vi "DefenderNormalNova.vi"(0 "Tipo de \nmarcador":T1(ring), 1 "Atacando contra?":bool=TRUE, 3 "AI Parameters":T9={"GotoKick"={"Dist do cone a frente"=150.0, "attacker farback"=1500.0, "Perto"=300.0, "min dist to kick"=150.0, "kick eps"=0.0, "Time to transition"=0.05}, "Attacker"={"CC chute"=0.09, "CC passe"=0.045, "Kick Force"=100.0, "ball-robot Kick"=200.0, "ball-robot Pass"=0.3, "drible\nAttk"=FALSE}, "Defender"={"D max"=1700.0, "Vel p/ robô av"=1000.0, "Kick Force"=100.0, "D atk-def"=0.0, "D farback"=0.0, "drible\ndef"=FALSE, "drible\ngoalie"=FALSE}, "Timeout"={"Field/v in x"=6.0, "Dist Robots"=300, "Dist up in y"=300}, "Pose Striker"={"dist"=200.0, "Numeric"=-4.0, "dist 2"=200.0, "drible\nstriker"=FALSE}, "Dist Stop"=300.0, "D ball out"=200, "D central gap "=150.0, "T pass"=0.0, "Force ++"=0.0, "range kick"=0.0, "Chute alto"=TRUE, "Marcador novo"=TRUE, "drible"=FALSE, "D drible"=300.0, "Versão Striker"=enum."Auto", "Defesa"=enum."Barreira", "Marcador"=enum."Marcar Segundo mais perigoso", "Receptor passe"=enum."Auto", "Área"=enum."Quadrada"} {"D drible" format="%#_13g"; "D central gap" format="%#_13g"; "Dist Stop" format="%#_13g"; "Pose Striker"."Numeric" format="%#_13g"; "Defender"."Kick Force" format="%#_13g"; "Defender"."Vel p/ robô av" format="%#_13g"; "Attacker"."ball-robot Kick" format="%#_13g"; "Attacker"."Kick Force" format="%#_13g"; "Attacker"."CC passe" format="%#_13g"; "Attacker"."CC chute" format="%#_13g"; "GotoKick"."kick eps" format="%#_13g"; "GotoKick"."min dist to kick" format="%#_13g"; "GotoKick"."Perto" format="%#_13g"; "GotoKick"."attacker farback" format="%#_13g"; "GotoKick"."Dist do cone a frente" format="%#_13g"}, 4 "IA State Input 2":T10={"our_robots"=[], "enemy_robots"=[], "balls"=[], "geometry"={"line_width"=0, "field_length"=0, "field_width"=0, "boundary_width"=0, "referee_width"=0, "goal_width"=0, "goal_depth"=0, "goal_wall_width"=0, "center_circle_radius"=0, "defense_radius"=0, "defense_stretch"=0, "free_kick_from_defense_dist"=0, "penalty_spot_from_field_line_dist"=0, "penalty_line_from_spot_dist"=0}, "IA Judge"={"stage"="", "command"="", "our_goalie_id"=0.0, "enemy_goalie_id"=0.0, "command enum"=enum."Halt", "Time"=enum."Azul"}, "Received Timestamp"=timestamp(0 s since 1904-01-01), "Events"={"Touch"=FALSE, "Ball out"=FALSE, "id touch"=0.0, "Ball out of \nVision"=FALSE, "Ball inside \nGoalie area"=FALSE, "Robot not responding"=FALSE, "Robots responding status"=[1.0, 1.0, 1.0, 1.0, 1.0, 1.0], "Enemy Ball \nPossession"=FALSE, "Pass State"=FALSE, "id end of pass"=0.0, "Kick"=FALSE, "Id ini Possession"=0.0, "Ball Possesion"=FALSE, "Id Possesion"=0.0, "Direct Kick"=FALSE, "2nd Strk Ativo"=FALSE}}, 5 "Stop?":bool, 6 "Defensores":u32[](array[numeric]), 7 "total de \ndefensores":i32, 8 "Field defense":dbl[](array[numeric]), 9 "geometry":T7, 10 "balls":T8[](array[typedef]), 11 "Our Robot":T2={"id"=0, "function"=enum."Attacker", "x"=0.0, "y"=0.0, "orientation"=0.0, "v_tangent"=0.0, "v_normal"=0.0, "v_ang"=0.0, "kick_x"=0.0, "kick_z"=0.0, "dribble"=FALSE, "Timestamp"=timestamp(0 s since 1904-01-01), "estimatives"={"est_v_tangent"=0.0, "est_v_normal"=0.0, "est_vx"=0.0, "est_vy"=0.0, "Pos Robot Est"=[]}, "dest_x_kick"=0.0, "dest_y_kick"=0.0, "Gap Coord"=[], "States"=enum."GoToTangent", "Path "=[], "Path  Smooth"=[], "Dest"=[]}) -> (2 "Robot out":T2={"id"=0, "function"=enum."Attacker", "x"=0.0, "y"=0.0, "orientation"=0.0, "v_tangent"=0.0, "v_normal"=0.0, "v_ang"=0.0, "kick_x"=0.0, "kick_z"=0.0, "dribble"=FALSE, "Timestamp"=timestamp(0 s since 1904-01-01), "estimatives"={"est_v_tangent"=0.0, "est_v_normal"=0.0, "est_vx"=0.0, "est_vy"=0.0, "Pos Robot Est"=[]}, "dest_x_kick"=0.0, "dest_y_kick"=0.0, "Gap Coord"=[], "States"=enum."GoToTangent", "Path "=[], "Path  Smooth"=[], "Dest"=[]})   [LabVIEW 2017]
uses:
  Core/AI Robot.ctl
  Functions Enum.ctl
  AttackerStates.ctl
  Path Planning/RRT/PathDests.ctl
  Path Planning/RRT/PathDest.ctl
  Core/AI Input.ctl
  Core/AI Ball.ctl
  Core/Field Size.ctl
  Core/AI Judge.ctl
  Command Enum.ctl
  Util/Events/Events.ctl
  AI Parameters.ctl
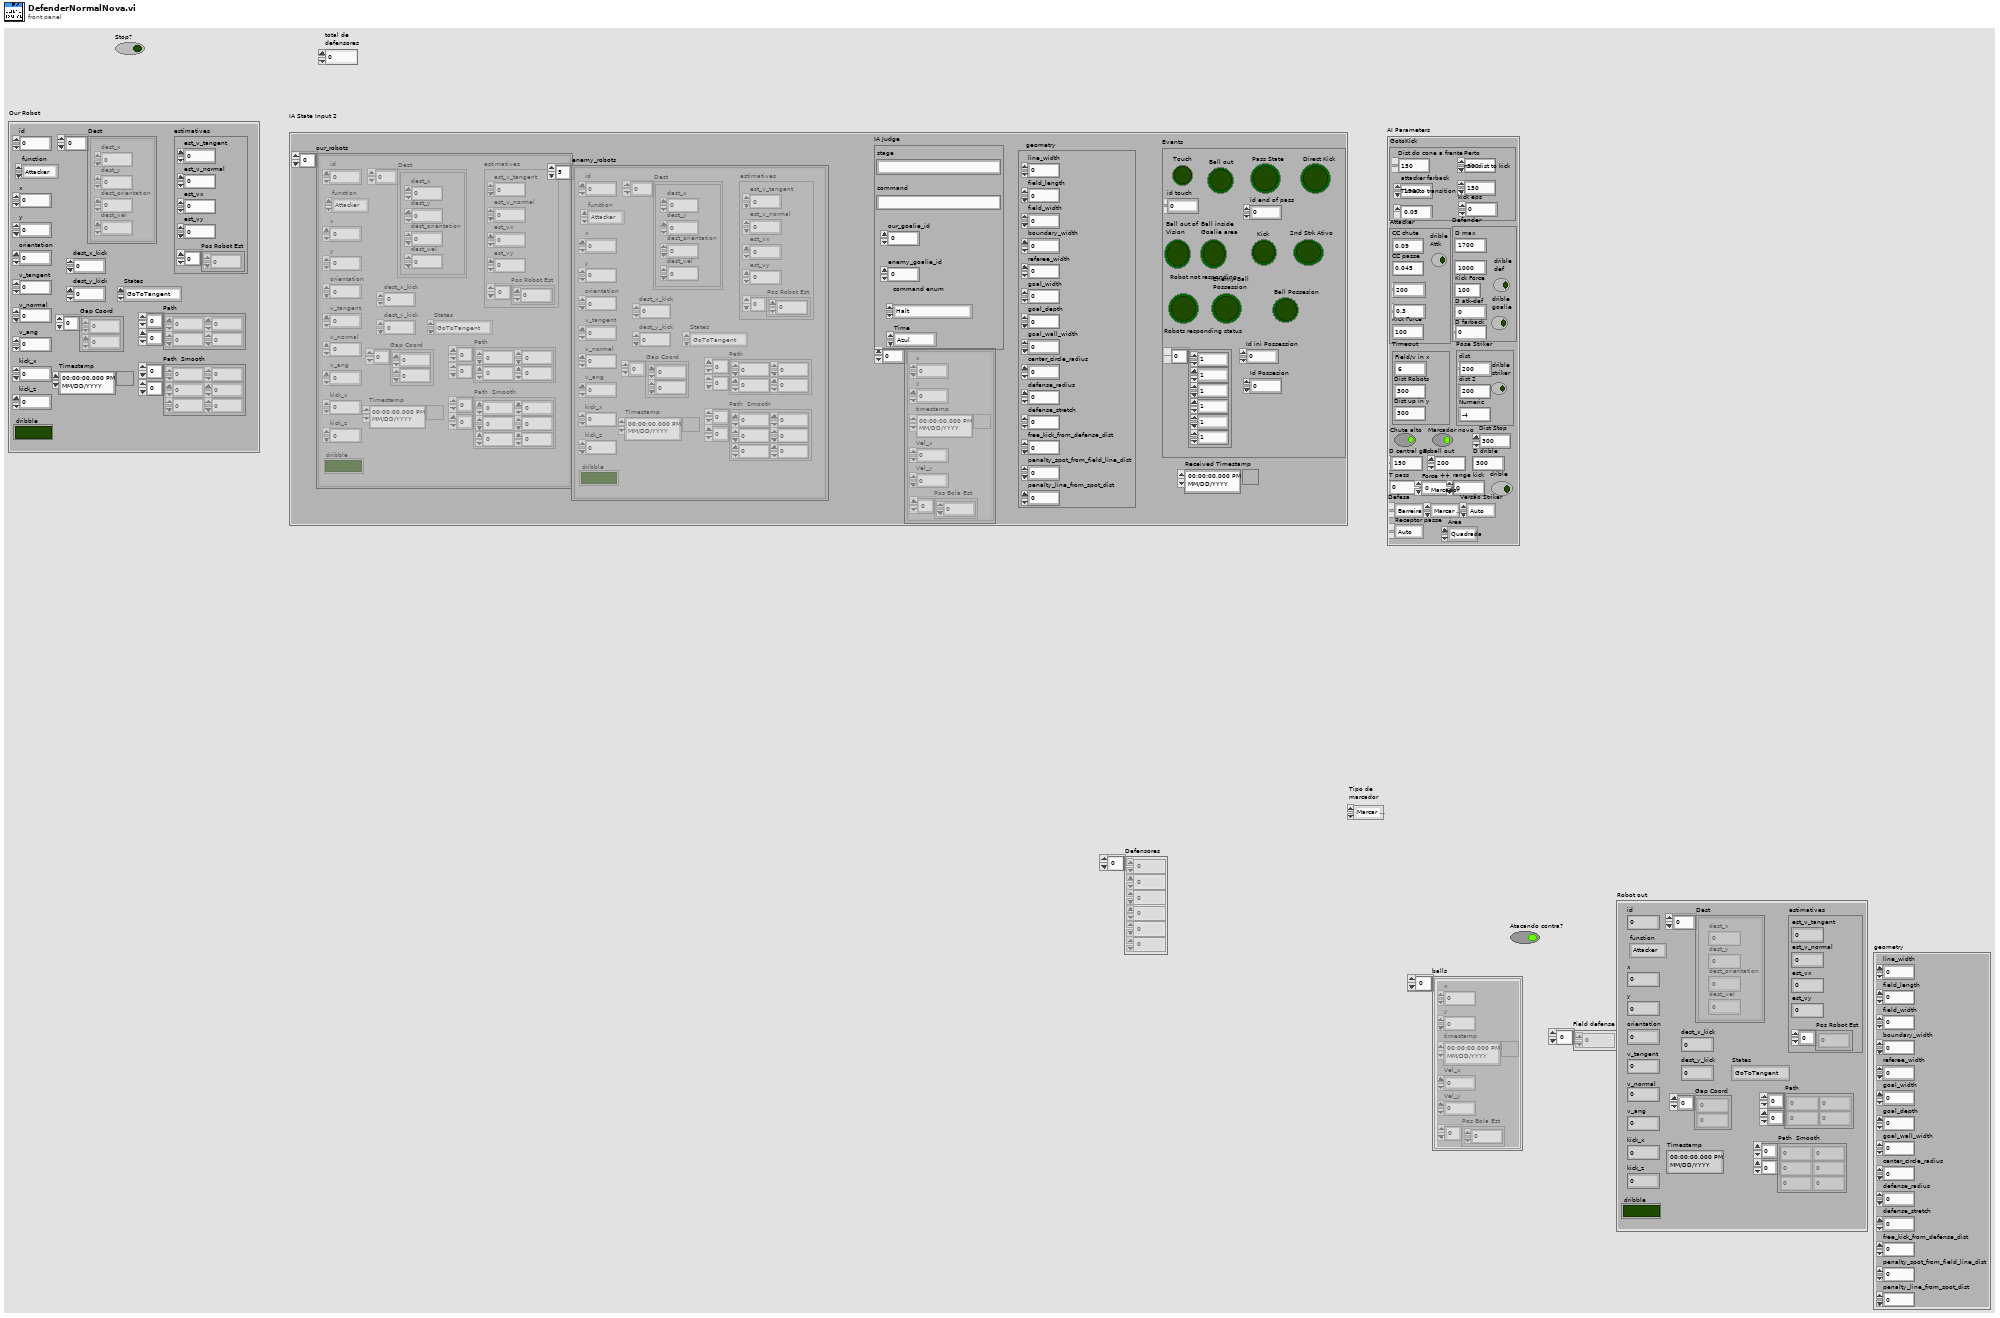
[diagram p1: front panel]
types:
  T1 = enum16{"Marcar Segundo mais perigoso", "Marcar o mais perigoso"}
  T2 = typedef "AI Robot.ctl" = cluster{"id":u32, "function":T3, "x":dbl, "y":dbl, "orientation":dbl, "v_tangent":dbl, "v_normal":dbl, "v_ang":dbl, "kick_x":dbl, "kick_z":dbl, "dribble":bool, "Timestamp":timestamp, "estimatives":cluster{"est_v_tangent":dbl, "est_v_normal":dbl, "est_vx":dbl, "est_vy":dbl, "Pos Robot Est":dbl[]}, "dest_x_kick":dbl, "dest_y_kick":dbl, "Gap Coord":dbl[], "States":T4, "Path ":dbl[][], "Path  Smooth":dbl[][], "Dest":T5}
  T3 = typedef "Functions Enum.ctl" = enum16{"2nd Striker", "Attacker", "Goalie", "Defender", "Striker", "Goto 0", "Dummy", "Kicker", "ZigZag 0", "ZigZag 1", "ZigZag 2", "ZigZag 3", "ZigZag 4", "ZigZag 5", "ZigZag 6", "ZigZag 7", "ZigZag 8", ""}
  T4 = typedef "AttackerStates.ctl" = enum16{"Pass", "GoToTangent", "BallGetting", "GoToKick", ""}
  T5 = typedef "PathDests.ctl" = T6[]
  T6 = typedef "PathDest.ctl" = cluster{"dest_x":dbl, "dest_y":dbl, "dest_orientation":dbl, "dest_vel":dbl}
  T7 = typedef "Field Size.ctl" = cluster{"line_width":u32, "field_length":u32, "field_width":u32, "boundary_width":u32, "referee_width":u32, "goal_width":u32, "goal_depth":u32, "goal_wall_width":u32, "center_circle_radius":u32, "defense_radius":u32, "defense_stretch":u32, "free_kick_from_defense_dist":u32, "penalty_spot_from_field_line_dist":u32, "penalty_line_from_spot_dist":u32}
  T8 = typedef "AI Ball.ctl" = cluster{"x":dbl, "y":dbl, "timestamp":timestamp, "Vel_x":dbl, "Vel_y":dbl, "Pos Bola Est":dbl[]}
  T9 = typedef "AI Parameters.ctl" = cluster{"GotoKick":cluster{"Dist do cone a frente":dbl, "attacker farback":dbl, "Perto":dbl, "min dist to kick":dbl, "kick eps":dbl, "Time to transition":dbl}, "Attacker":cluster{"CC chute":dbl, "CC passe":dbl, "Kick Force":dbl, "ball-robot Kick":dbl, "ball-robot Pass":dbl, "drible\nAttk":bool}, "Defender":cluster{"D max":dbl, "Vel p/ robô av":dbl, "Kick Force":dbl, "D atk-def":dbl, "D farback":dbl, "drible\ndef":bool, "drible\ngoalie":bool}, "Timeout":cluster{"Field/v in x":dbl, "Dist Robots":u32, "Dist up in y":u32}, "Pose Striker":cluster{"dist":dbl, "Numeric":dbl, "dist 2":dbl, "drible\nstriker":bool}, "Dist Stop":dbl, "D ball out":i32, "D central gap ":dbl, "T pass":dbl, "Force ++":dbl, "range kick":dbl, "Chute alto":bool, "Marcador novo":bool, "drible":bool, "D drible":dbl, "Versão Striker":enum16{"Auto", "3", "2", "1"}, "Defesa":enum16{"ManMark", "Barreira"}, "Marcador":enum16{"Marcar Segundo mais perigoso", "Marcar o mais perigoso"}, "Receptor passe":enum16{"Auto", "2nd Striker", "Striker"}, "Área":enum16{"Quadrada", "Circular"}}
  T10 = typedef "AI Input.ctl" = cluster{"our_robots":T2[], "enemy_robots":T2[], "balls":T8[], "geometry":T7, "IA Judge":T11, "Received Timestamp":timestamp, "Events":T13}
  T11 = typedef "AI Judge.ctl" = cluster{"stage":string, "command":string, "our_goalie_id":dbl, "enemy_goalie_id":dbl, "command enum":T12, "Time":enum16{"Azul", "Amarelo"}}
  T12 = typedef "Command Enum.ctl" = enum16{"Halt", "Stop", "Force Start", "PKA Normal Start", "Prepare Kickoff Ally", "PKE Normal Start", "Prepare Kickoff Enemy", "Prepare Penalty Ally", "PPA Normal Start", "Prepare Penalty Enemy", "PPE Normal Start", "Direct Free Enemy", "Direct Free Ally", "Indirect Free Enemy", "Indirect Free Ally", "Timeout Enemy", "Timeout Ally", "Goal Enemy", "Goal Ally", "Ball Placement Enemy", "Ball Placement Ally", "Normal Half Time", "Extra Time Break", "Extra Half Time", "None", "Post Game"}
  T13 = typedef "Events.ctl" = cluster{"Touch":bool, "Ball out":bool, "id touch":dbl, "Ball out of \nVision":bool, "Ball inside \nGoalie area":bool, "Robot not responding":bool, "Robots responding status":dbl[], "Enemy Ball \nPossession":bool, "Pass State":bool, "id end of pass":dbl, "Kick":bool, "Id ini Possession":dbl, "Ball Possesion":bool, "Id Possesion":dbl, "Direct Kick":bool, "2nd Strk Ativo":bool}
  T14 = typedef "AI Robot.ctl" = cluster{"id":u32, "function":T15, "x":dbl, "y":dbl, "orientation":dbl, "v_tangent":dbl, "v_normal":dbl, "v_ang":dbl, "kick_x":dbl, "kick_z":dbl, "dribble":bool, "Timestamp":timestamp, "estimatives":cluster{"est_v_tangent":dbl, "est_v_normal":dbl, "est_vx":dbl, "est_vy":dbl, "Pos Robot Est":dbl[]}, "dest_x_kick":dbl, "dest_y_kick":dbl, "Gap Coord":dbl[], "States":T4, "Path ":dbl[][], "Path  Smooth":dbl[][], "Dest":T5}
  T15 = typedef "Functions Enum.ctl" = enum16{"Attacker", "Goalie", "Defender", "Striker", "Goto 0", "Dummy", "Kicker", "ZigZag"}
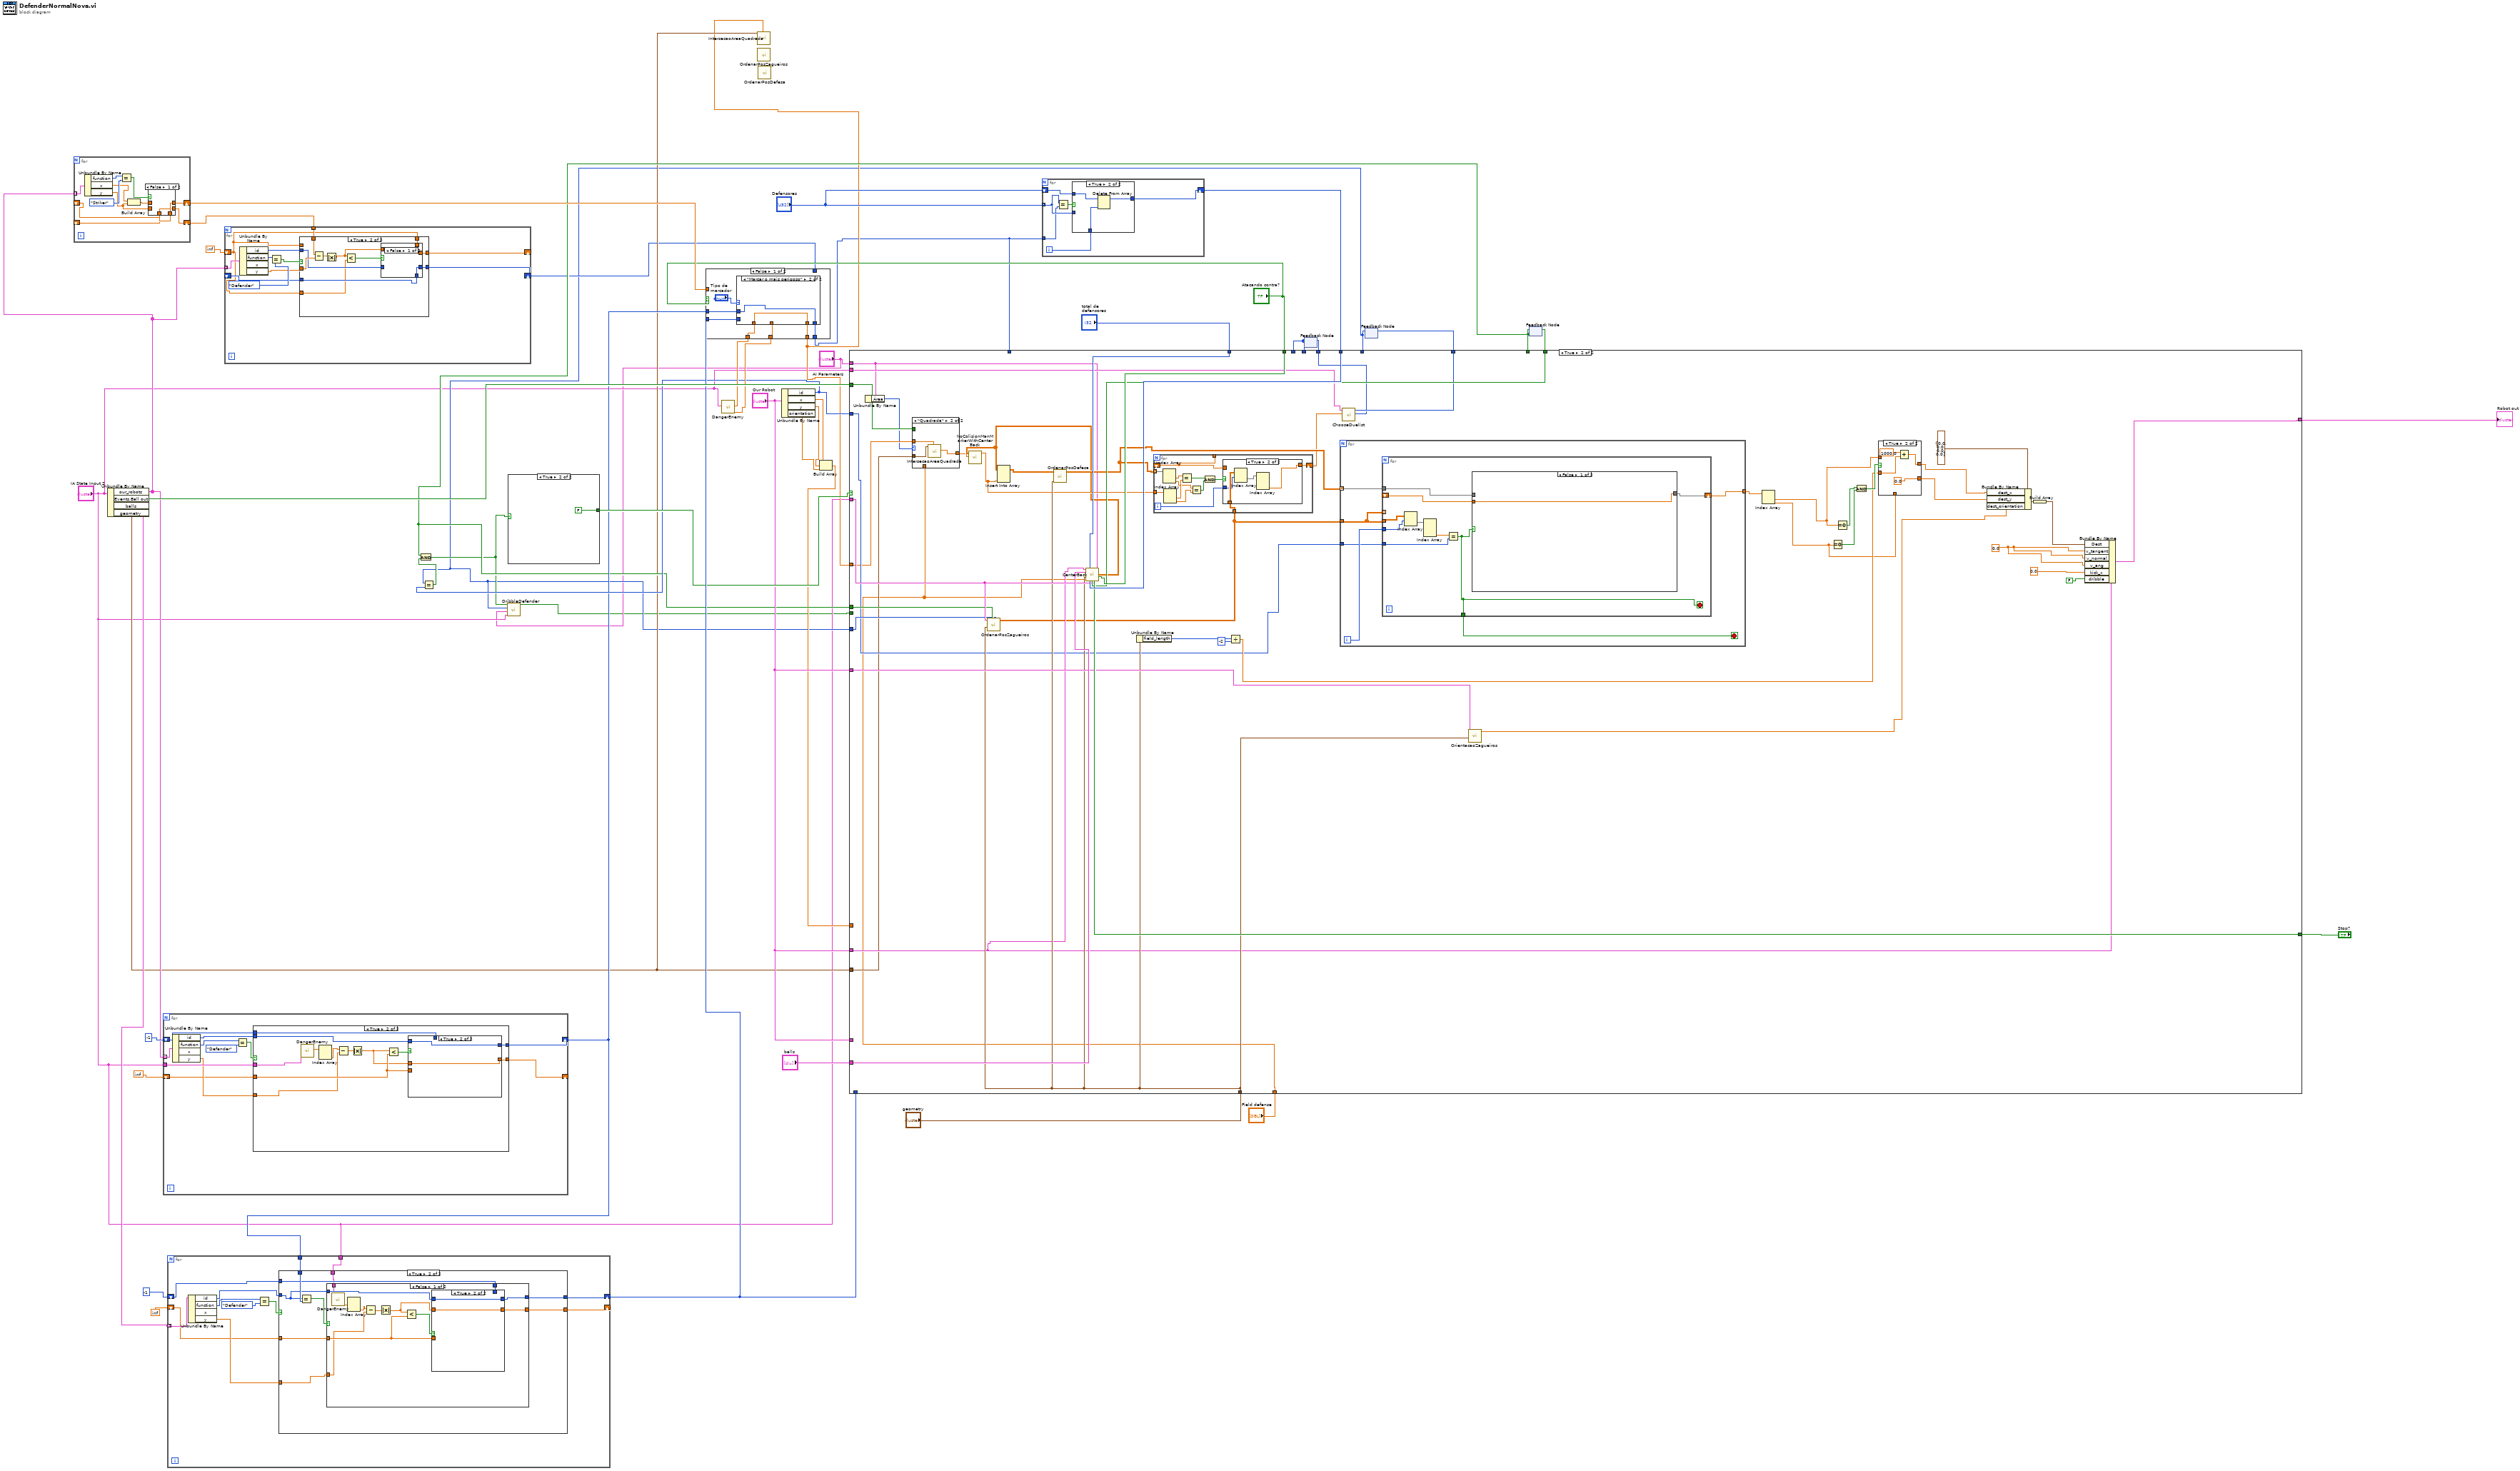
[diagram p0: block diagram]
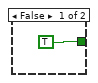
[diagram p2: hidden frame]
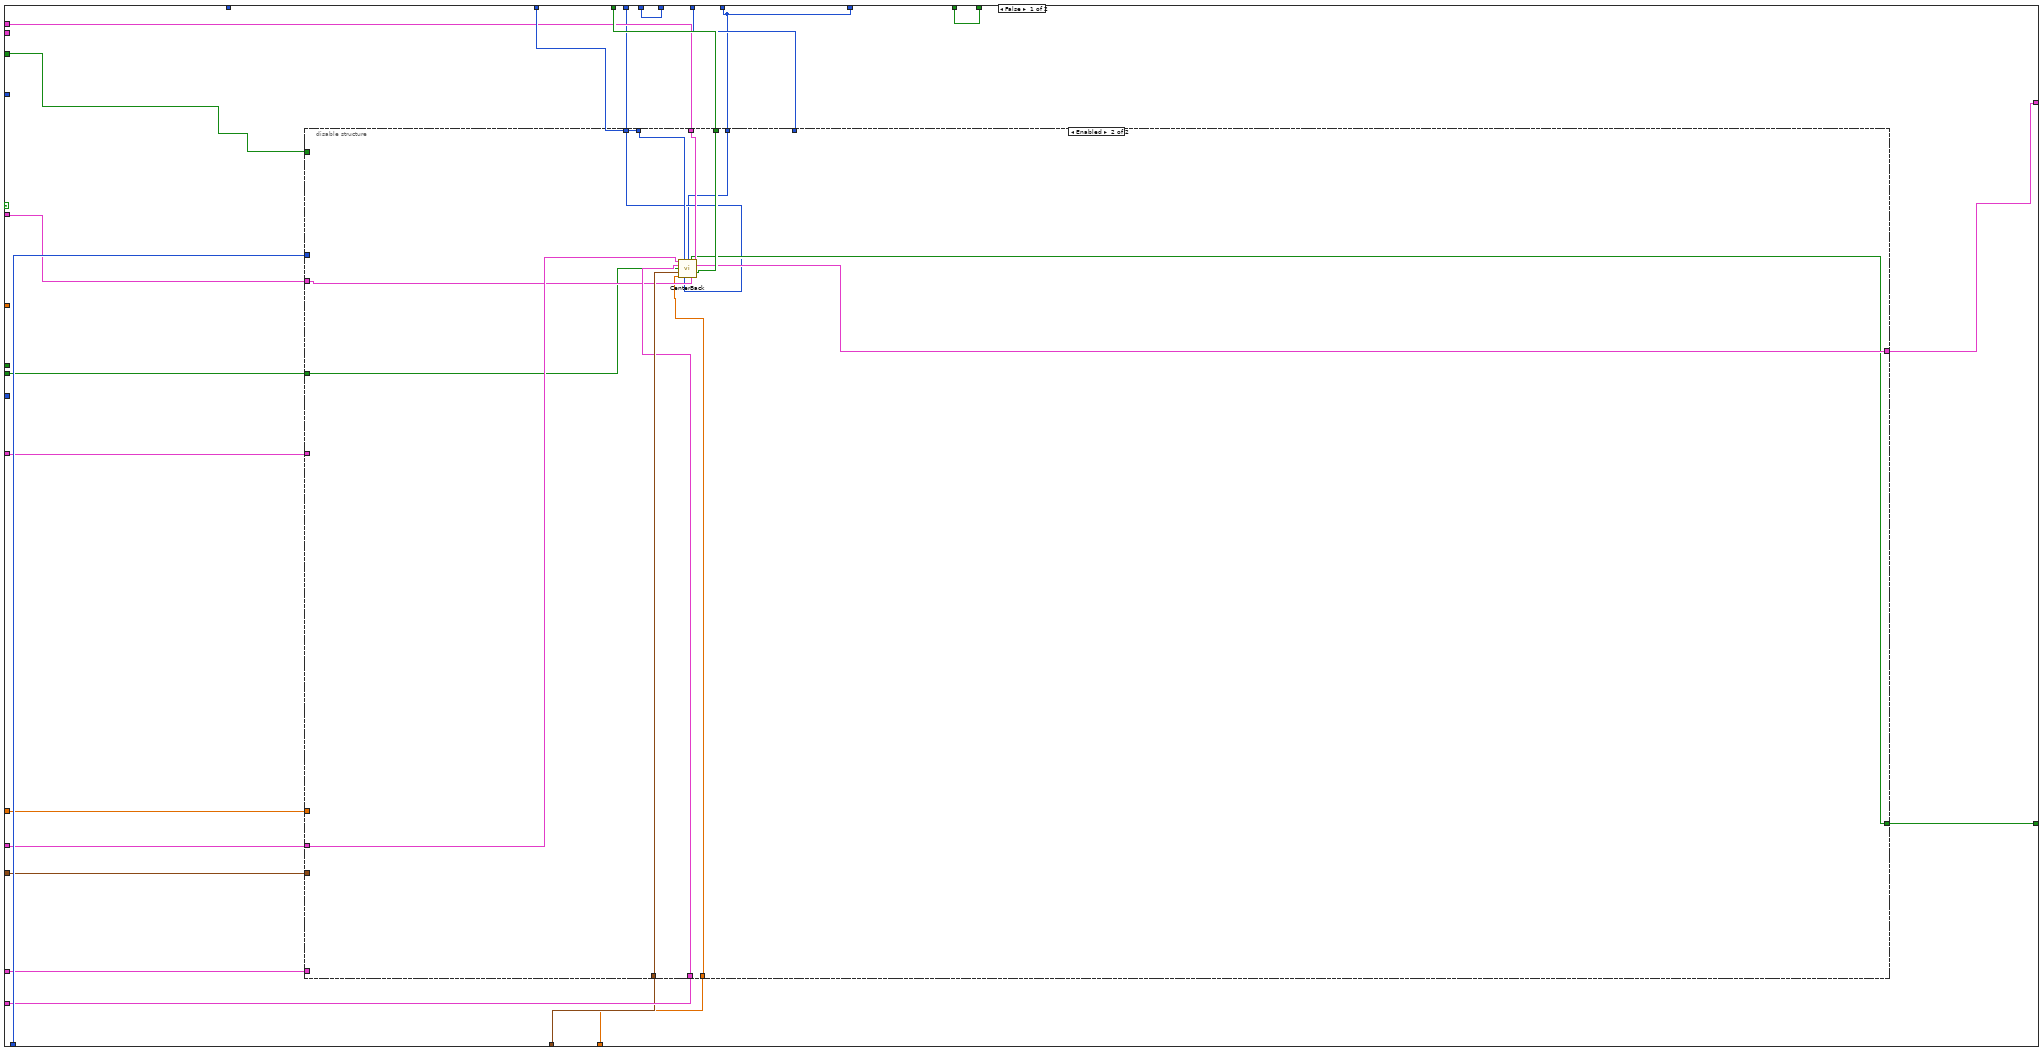
[diagram p12: hidden frame]
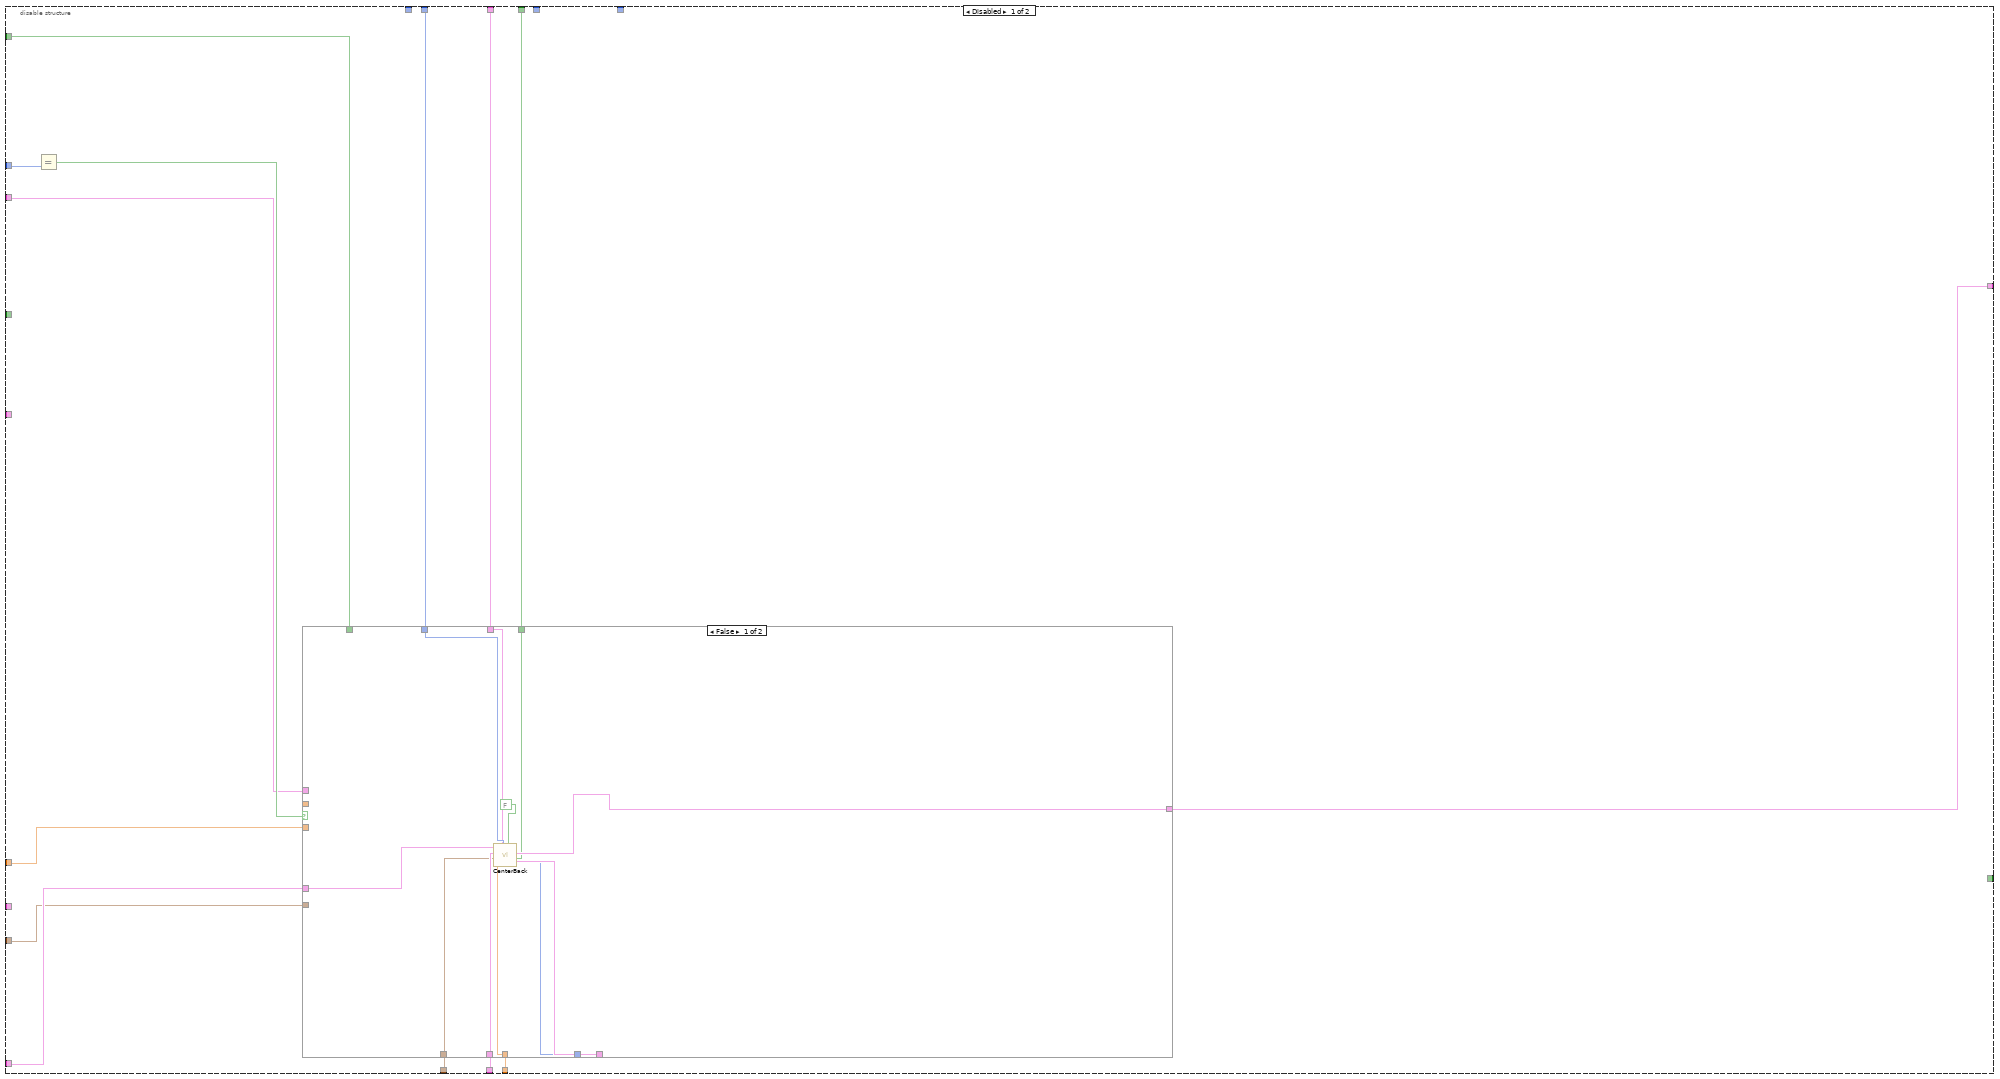
[diagram p13: hidden frame]
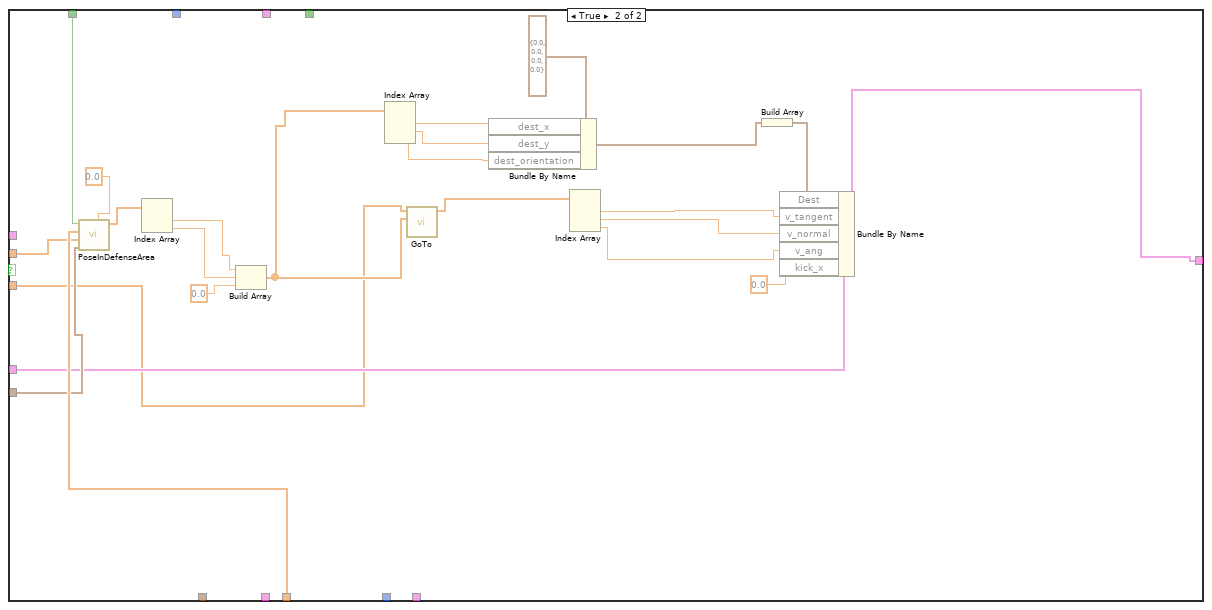
[diagram p14: hidden frame]
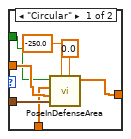
[diagram p15: hidden frame]
diagram:
  n1 = Unbundle By Name("IA State Input 2") -> ("our_robots"=w18:T2[], "Events.Ball out"=w40:bool, "geometry"=w11:T7)  [unwired: 1 out]
  n2 = for {
    tunnel: w18 -> [w55] mode=indexing
    shift-right: [w49] -> w34
    shift-left: _ -> [w48]
    shift-right: [w46] -> w25
    shift-left: _ -> [w45]
    n3 = Unbundle By Name(w55) -> ("function"=w54:T3, "x"=w51:dbl, "y"=w47:dbl)
    n4 = Equal?(x=w54, y=Functions_Enum."Striker" ("x")) -> (x = y?=w52:bool)
    n5 = Build Array(w51, w47) -> (w50:dbl[])
    n6 = case shown="False" w52 {
      tunnel: w50 -> [_ w59]
      tunnel: [w57 w59] -> w49
      tunnel: w48 -> [w57 _]
      tunnel: [w56 w58] -> w46
      tunnel: w47 -> [_ w58]
      tunnel: w45 -> [w56 _]
      frame False {
      }
      frame True {
      }
    }
  }
  n7 = for {
    tunnel: w18 -> [w70] mode=indexing
    tunnel: "IA State Input 2" -> [w66]
    shift-right: [w63] -> w17
    shift-left: -1 -> [w60]
    shift-right: [w62] -> _
    shift-left: inf -> [w61]
    n8 = Unbundle By Name(w70) -> ("id"=w64:u32, "function"=w69:T3, "y"=w65:dbl)  [unwired: 1 out]
    n9 = Equal?(x=w69, y=Functions_Enum."Defender" ("x")) -> (x = y?=w67:bool)
    n10 = case shown="True" w67 {
      tunnel: w66 -> [_ w84]
      tunnel: w65 -> [_ w75]
      tunnel: w64 -> [_ w82]
      tunnel: [w72 w81] -> w63
      tunnel: [w71 w80] -> w62
      tunnel: w61 -> [w71 w79]
      tunnel: w60 -> [w72 w78]
      frame False {
      }
      frame True {
        n11 = call "DangerEnemy.vi"("IA Input"=w84) -> ("Pos do inimigo\nperigoso"=w77:dbl[])  [unwired: 5 in, 5 out]
        n12 = Index Array(array=w77) -> (element #2=w76:dbl)  [unwired: 2 in, 1 out]
        n13 = Subtract(x=w76, y=w75) -> (x-y=w74:dbl)
        n14 = Absolute Value(x=w74) -> (abs(x)=w73:dbl)
        n15 = Less?(x=w73, y=w79) -> (x < y?=w83:bool)
        n16 = case shown="True" w83 {
          tunnel: w82 -> [_ w88]
          tunnel: [w85 w88] -> w81
          tunnel: [w86 w87] -> w80
          tunnel: w73 -> [_ w87]
          tunnel: w79 -> [w86 _]
          tunnel: w78 -> [w85 _]
          frame False {
          }
          frame True {
          }
        }
      }
    }
  }
  n17 = for {
    tunnel: w18 -> [w100] mode=indexing
    tunnel: w17 -> [w97]
    shift-right: [w95] -> _
    shift-left: inf -> [w92]
    shift-right: [w94] -> w35
    shift-left: -1 -> [w93]
    tunnel: "IA State Input 2" -> [w91]
    n18 = Unbundle By Name(w100) -> ("id"=w89:u32, "function"=w90:T3, "y"=w96:dbl)  [unwired: 1 out]
    n19 = Equal?(x=w90, y=Functions_Enum."Defender" ("x")) -> (x = y?=w98:bool)
    n20 = case shown="True" w98 {
      tunnel: w89 -> [_ w107]
      tunnel: w97 -> [_ w111]
      tunnel: w96 -> [_ w104]
      tunnel: [w101 w109] -> w95
      tunnel: [w102 w108] -> w94
      tunnel: w93 -> [w102 w106]
      tunnel: w92 -> [w101 w105]
      tunnel: w91 -> [_ w103]
      frame False {
      }
      frame True {
        n21 = Equal?(x=w107, y=w111) -> (x = y?=w110:bool)
        n22 = case shown="False" w110 {
          tunnel: w104 -> [w114 _]
          tunnel: [w122 w128] -> w109
          tunnel: [w120 w129] -> w108
          tunnel: w107 -> [w121 _]
          tunnel: w106 -> [w119 w129]
          tunnel: w105 -> [w118 w128]
          tunnel: w103 -> [w117 _]
          frame False {
            n23 = call "DangerEnemy.vi"("IA Input"=w117) -> ("Pos do segundo inimigo\nperigoso"=w116:dbl[])  [unwired: 5 in, 5 out]
            n24 = Index Array(array=w116) -> (element #2=w115:dbl)  [unwired: 2 in, 1 out]
            n25 = Subtract(x=w115, y=w114) -> (x-y=w113:dbl)
            n26 = Absolute Value(x=w113) -> (abs(x)=w112:dbl)
            n27 = Less?(x=w112, y=w118) -> (x < y?=w123:bool)
            n28 = case shown="True" w123 {
              tunnel: [w124 w127] -> w122
              tunnel: w112 -> [_ w127]
              tunnel: [w125 w126] -> w120
              tunnel: w121 -> [_ w126]
              tunnel: w119 -> [w125 _]
              tunnel: w118 -> [w124 _]
              frame False {
              }
              frame True {
              }
            }
          }
          frame True {
          }
        }
      }
    }
  }
  n29 = for {
    tunnel: w18 -> [w140] mode=indexing
    tunnel: w25 -> [w136]
    shift-right: [w135] -> _
    shift-left: inf -> [w131]
    shift-right: [w133] -> w9
    shift-left: _ -> [w132]
    n30 = Unbundle By Name(w140) -> ("id"=w134:u32, "function"=w139:T3, "y"=w130:dbl)  [unwired: 1 out]
    n31 = Equal?(x=w139, y=Functions_Enum."Defender") -> (x = y?=w137:bool)
    n32 = case shown="True" w137 {
      tunnel: w130 -> [_ w153]
      tunnel: w136 -> [_ w152]
      tunnel: [w142 w150] -> w135
      tunnel: w134 -> [_ w149]
      tunnel: [w141 w148] -> w133
      tunnel: w132 -> [w141 w147]
      tunnel: w131 -> [_ w146]
      tunnel: w131 -> [w142 _]
      tunnel: w131 -> [_ w145]
      frame False {
      }
      frame True {
        n33 = Subtract(x=w152, y=w153) -> (x-y=w144:dbl)
        n34 = Absolute Value(x=w144) -> (abs(x)=w143:dbl)
        n35 = Less?(x=w143, y=w145) -> (x < y?=w151:bool)
        n36 = case shown="False" w151 {
          tunnel: w143 -> [_ w157]
          tunnel: [w154 w157] -> w150
          tunnel: w149 -> [_ w156]
          tunnel: [w155 w156] -> w148
          tunnel: w147 -> [w155 _]
          tunnel: w146 -> [w154 _]
          frame False {
          }
          frame True {
          }
        }
      }
    }
  }
  n37 = call "DangerEnemy.vi"("IA Input"="IA State Input 2") -> ("Pos do segundo inimigo\nperigoso"=w37:dbl[], "Pos do inimigo\nperigoso"=w38:dbl[])  [unwired: 5 in, 4 out]
  n38 = case shown="False" "Atacando contra?" {
    tunnel: w34 -> [_ w170]
    tunnel: [w163 w170] -> w10
    tunnel: w38 -> [w164 _]
    tunnel: w37 -> [w162 _]
    tunnel: w17 -> [w161 _]
    tunnel: [w160 w169] -> w8
    tunnel: w35 -> [w159 _]
    tunnel: w9 -> [_ w169]
    frame False {
      n39 = case shown="\"Marcar o mais perigoso\"" "Tipo de \nmarcador" {
        tunnel: w164 -> [_ w167]
        tunnel: [w165 w167] -> w163
        tunnel: w162 -> [w165 _]
        tunnel: [w166 w168] -> w160
        tunnel: w161 -> [_ w168]
        tunnel: w159 -> [w166 _]
        frame "Marcar Segundo mais perigoso" {
        }
        frame "Marcar o mais perigoso" {
        }
      }
    }
    frame True {
    }
  }
  n40 = call "IntersecaoAreaQuadrada.vi"("Pos entrada"=w10, "geometry"=w11) -> ()  [unwired: 8 in, 2 out]
  n41 = call "OrdenarPosZagueiros.vi"() -> ()  [unwired: 11 in, 1 out]
  n42 = call "OrdenarPosDefesa.vi"() -> ()  [unwired: 11 in, 1 out]
  n43 = Unbundle By Name("Our Robot") -> ("id"=w19:u32, "x"=w15:dbl, "y"=w14:dbl, "orientation"=w13:dbl)
  n44 = Build Array(w15, w14, w13) -> (w12:dbl[])
  n45 = for {
    tunnel: "Defensores" -> [w172] mode=indexing
    tunnel: w8 -> [w171]
    shift-right: [w174] -> w32
    shift-left: "Defensores" -> [w173]
    i -> [w175]
    n46 = Equal?(x=w172, y=w171) -> (x = y?=w176:bool)
    n47 = case shown="True" w176 {
      tunnel: w173 -> [w177 w179]
      tunnel: w175 -> [_ w178]
      tunnel: [w177 w180] -> w174
      tunnel: w172 -> [_ _]
      frame False {
      }
      frame True {
        n48 = Delete From Array(array=w179, index=w178) -> (array with subset deleted=w180:u32[])  [unwired: 1 in, 1 out]
      }
    }
  }
  n49 = feedback #1() -> (w6:u32[])  [unwired: 1 in]
  n50 = feedback #2() -> (w4:u32)  [unwired: 1 in]
  n51 = Equal?(x=w4, y=w19) -> (x = y?=w28:bool)
  n52 = feedback #3() -> (w16:bool)  [unwired: 1 in]
  n53 = And(x=w16, y=w28) -> (x .and. y?=w5:bool)
  n54 = call "DribbleDefender.vi"("IA State Input 2"="IA State Input 2", "AI Parameters"="AI Parameters", "Id duelist"=w4, "Id duelist atuando?"=w5) -> ("Dribble?"=w1:bool)  [unwired: 7 in]
  n55 = case shown="True" w5 {
    tunnel: [TRUE FALSE] -> w27
    frame False {
    }
    frame True {
    }
  }
  n56 = case shown="True" w27 {
    tunnel: "IA State Input 2" -> [w202 w307]
    tunnel: "Our Robot" -> [w203 _]
    tunnel: w19 -> [_ w288]
    tunnel: w35 -> [w204 _]
    tunnel: [w191 w296] -> w26
    tunnel: w11 -> [w200 w275]
    tunnel: w40 -> [w201 w271]
    tunnel: w12 -> [w199 _]
    tunnel: "Our Robot" -> [w193 w297]
    tunnel: w10 -> [_ w274]
    tunnel: "total de \ndefensores" -> [w198 w313]
    tunnel: "Atacando contra?" -> [w197 w315]
    tunnel: "AI Parameters" -> [w196 w270]
    tunnel: "balls" -> [w195 w316]
    tunnel: "geometry" -> [w194 w306]
    tunnel: "Field defense" -> [w192 w272]
    tunnel: "Stop?" -> [w190 w312]
    tunnel: w32 -> [w189 w314]
    tunnel: [w184 w282] -> w30
    tunnel: w4 -> [w184 _]
    tunnel: [w187 w310] -> w29
    tunnel: w16 -> [w187 _]
    tunnel: "Our Robot" -> [w188 w311]
    tunnel: w16 -> [_ w304]
    tunnel: w4 -> [_ w303]
    tunnel: w8 -> [_ _]
    tunnel: "IA State Input 2" -> [_ w280]
    tunnel: [w186 w279] -> w7
    tunnel: w6 -> [w186 _]
    tunnel: w6 -> [w185 _]
    tunnel: w1 -> [w183 _]
    frame False {
      n57 = disable-structure shown="Enabled" {
        disable-tunnel: w204 -> [w219 _]
        disable-tunnel: w203 -> [w217 _]
        disable-tunnel: w202 -> [w216 w265]
        disable-tunnel: [w215 w261] -> w191
        disable-tunnel: w192 -> [w214 w258]
        disable-tunnel: w201 -> [w213 _]
        disable-tunnel: w200 -> [w212 _]
        disable-tunnel: w199 -> [w210 _]
        disable-tunnel: w198 -> [w209 w263]
        disable-tunnel: w197 -> [w208 w264]
        disable-tunnel: w196 -> [w207 w262]
        disable-tunnel: w195 -> [w206 w266]
        disable-tunnel: w194 -> [w205 w267]
        disable-tunnel: w193 -> [_ w268]
        disable-tunnel: w190 -> [_ w260]
        disable-tunnel: w189 -> [_ _]
        disable-tunnel: w188 -> [_ _]
        disable-tunnel: w185 -> [_ w259]
        disable-tunnel: w184 -> [_ w257]
        disable-tunnel: w183 -> [_ w256]
        frame Disabled {
          n58 = Equal?(y=w219) -> (x=w220:u32, x = y?=w218:bool)
          n59 = case shown="False" w218 {
            tunnel: _ -> [w230 _]
            tunnel: w217 -> [w229 w235]
            tunnel: w216 -> [_ _]
            tunnel: [w228 w233] -> w215
            tunnel: w214 -> [w227 w254]
            tunnel: w213 -> [_ w255]
            tunnel: w212 -> [_ w253]
            tunnel: [_ w252] -> w211
            tunnel: w210 -> [_ w234]
            tunnel: w209 -> [w226 _]
            tunnel: w208 -> [w225 _]
            tunnel: w207 -> [w224 _]
            tunnel: w206 -> [w223 _]
            tunnel: w205 -> [w222 _]
            tunnel: _ -> [w221 _]
            frame False {
              n60 = call "CenterBack.vi"("Atacando contra?"=w225, "AI Parameters"=w224, "IA State Input 2"=w230, "Stop?"=FALSE, "Defensores"=w221, "total"=w226, "Field defense"=w227, "Field Size in"=w222, "balls"=w223, "Our Robot in"=w229) -> ("Robot out"=w228:T14)  [unwired: 1 in]
            }
            frame True {
              n61 = call "PoseInDefenseArea.vi"("theta"=0.0, "geometry"=w253, "Ball"=w252, "Field defense"=w254, "Events.Ball out"=w255) -> ("Array"=w238:dbl[])  [unwired: 6 in]
              n62 = Index Array(array=w238) -> (element #1=w237:dbl, element #2=w236:dbl)  [unwired: 2 in]
              n63 = Build Array(w237, w236, 0.0 ("element")) -> (w249:dbl[])
              n64 = Index Array(array=w249) -> (element #1=w247:dbl, element #2=w246:dbl, element #3=w245:dbl)  [unwired: 3 in]
              n65 = call "GoTo.vi"("Target"=w249, "Position"=w234) -> ("Output\nVelocity"=w250:dbl[])  [unwired: 8 in, 1 out]
              n66 = Bundle By Name(cluster=T6 {"dest_x"=0.0, "dest_y"=0.0, "dest_orientation"=0.0, "dest_vel"=0.0} ("element"), "dest_x"=w247, "dest_y"=w246, "dest_orientation"=w245) -> (w243:T6)
              n67 = Index Array(array=w250) -> (element #1=w242:dbl, element #2=w241:dbl, element #3=w240:dbl)  [unwired: 3 in]
              n68 = Build Array(w243) -> (w244:T6[])
              n69 = Bundle By Name(cluster=w235, "Dest"=w244, "v_tangent"=w242, "v_normal"=w241, "v_ang"=w240, "kick_x"=0.0) -> (w233:T2)
            }
          }
        }
        frame Enabled {
          n70 = call "CenterBack.vi"("Our Robot in"=w268, "total"=w263, "Id duelist"=w257, "Stop?"=w260, "AI Parameters"=w262, "balls"=w266, "Dribble"=w256, "Field Size in"=w267, "Atacando contra?"=w264, "Field defense"=w258, "Defensores"=w259, "IA State Input 2"=w265) -> ("Robot out"=w261:T2)  [unwired: 1 in, 2 out]
        }
      }
    }
    frame True {
      w298 = 0.0
      n71 = Unbundle By Name(w270) -> ("Área"=w269:enum16{"Quadrada", "Circular"})
      n72 = case shown="\"Quadrada\"" w269 {
        tunnel: w275 -> [w320 w326]
        tunnel: w274 -> [w319 w325]
        tunnel: [w323 w324] -> w273
        tunnel: w272 -> [w318 _]
        tunnel: w271 -> [w317 _]
        frame "Circular" {
          n73 = call "PoseInDefenseArea.vi"("theta"=0.0, "Recuo"=-250.0, "geometry"=w320, "Ball"=w319, "Field defense"=w318, "Events.Ball out"=w317) -> ("Array"=w323:dbl[])  [unwired: 5 in]
        }
        frame "Quadrada" {
          n74 = call "IntersecaoAreaQuadrada.vi"("Pos entrada"=w325, "geometry"=w326) -> ("Pos de Interseção"=w324:dbl[])  [unwired: 8 in, 1 out]
        }
      }
      n75 = call "OrdenarPosZagueiros.vi"("ID duelist"=w303, "Zagueiro duelist?"=w304, "geometry"=w306, "IA State Input 2"=w307) -> ("Posições ordenadas zagueiros"=w283:dbl[][])  [unwired: 7 in]
      n76 = call "CenterBack.vi"("Our Robot in"=w297, "total"=w313, "Stop?"=w312, "AI Parameters"=w270, "balls"=w316, "Field Size in"=w306, "Atacando contra?"=w315, "Field defense"=w272, "Defensores"=w314, "IA State Input 2"=w307) -> ("Pos Centers Back"=w276:dbl[][], "Zageuiro duelist?"=w310:bool)  [unwired: 3 in, 1 out]
      n77 = call "NoColisionManMarkerWithCenterBack.vi"("Pos ManMarker"=w273, "Pos CenterBacks"=w276) -> ("Pos ManMarker"=w277:dbl[])  [unwired: 9 in]
      n78 = Insert Into Array(array=w276, new element=w277) -> (w305:dbl[][])  [unwired: 2 in]
      n79 = call "OrdenarPosDefesa.vi"("geometry"=w306, "Posições da defesa"=w305) -> ("Posições ordenadas"=w284:dbl[][])  [unwired: 9 in]
      n80 = Unbundle By Name(w306) -> ("field_length"=w309:u32)
      n81 = for {
        tunnel: w284 -> [w339] mode=indexing
        tunnel: w277 -> [w338]
        tunnel: w283 -> [w330]
        shift-right: [w329] -> w281
        shift-left: _ -> [w328]
        tunnel: [w328] -> _
        i -> [w327]
        n82 = Index Array(array=w339) -> (element #1=w337:dbl, element #2=w335:dbl)  [unwired: 2 in]
        n83 = Index Array(array=w338) -> (element #1=w336:dbl, element #2=w334:dbl)  [unwired: 2 in]
        n84 = Equal?(x=w337, y=w336) -> (x = y?=w333:bool)
        n85 = Equal?(x=w335, y=w334) -> (x = y?=w332:bool)
        n86 = And(x=w333, y=w332) -> (x .and. y?=w331:bool)
        n87 = case shown="True" w331 {
          tunnel: w330 -> [_ w344]
          tunnel: w327 -> [_ w343]
          tunnel: [w340 w341] -> w329
          tunnel: w328 -> [w340 _]
          frame False {
          }
          frame True {
            n88 = Index Array(array=w344, index (row)=w343) -> (element=w342:dbl[])  [unwired: 1 in]
            n89 = Index Array(array=w342) -> (element #3=w341:dbl)  [unwired: 3 in, 2 out]
          }
        }
      }
      n90 = Divide(x=w309, y=-2) -> (x/y=w289:dbl)
      n91 = for {
        tunnel: w284 -> [w348] mode=indexing
        tunnel: w283 -> [w345]
        tunnel: w288 -> [w349]
        tunnel: [w347] -> w287
        i -> [w350]
        stop <- w346 stop-if-true
        n92 = for {
          tunnel: w345 -> [w359]
          tunnel: w350 -> [w358]
          tunnel: w349 -> [w355]
          tunnel: w348 -> [w354]
          shift-right: [w353] -> w347
          shift-left: _ -> [w352]
          tunnel: [w351] -> w346
          tunnel: w345 -> [_] mode=indexing
          stop <- w351 stop-if-true
          n93 = Index Array(array=w359, index (row)=w358) -> (element=w357:dbl[])  [unwired: 1 in]
          n94 = Index Array(array=w357) -> (element #3=w356:dbl)  [unwired: 3 in, 2 out]
          n95 = Equal?(x=w356, y=w355) -> (x = y?=w351:bool)
          n96 = case shown="False" w351 {
            tunnel: [w360 w361] -> w353
            tunnel: w354 -> [_ w361]
            tunnel: w352 -> [w360 _]
            frame False {
            }
            frame True {
            }
          }
        }
      }
      n97 = call "ChooseDuelist.vi"("Id Manmarker"=w281, "IA State Input 2"=w280) -> ("Defensores 2"=w279:u32[], "Id Duelist"=w282:u32)  [unwired: 8 in]
      n98 = call "OrientacaoZagueiros.vi"("geometry"=w306, "Our Robot"=w311) -> ("Orientação Center Back"=w295:dbl)  [unwired: 9 in]
      n99 = Index Array(array=w287) -> (element #1=w286:dbl, element #2=w285:dbl)  [unwired: 2 in]
      n100 = Equal To 0?(x=w285) -> (x = 0?=w293:bool)
      n101 = Equal To 0?(x=w286) -> (x = 0?=w294:bool)
      n102 = And(x=w294, y=w293) -> (x .and. y?=w292:bool)
      n103 = case shown="True" w292 {
        tunnel: [w363 w365] -> w291
        tunnel: w286 -> [w363 _]
        tunnel: [w362 0.0] -> w290
        tunnel: w285 -> [w362 _]
        tunnel: w289 -> [_ w364]
        frame False {
        }
        frame True {
          n104 = Add(x=1000.0, y=w364) -> (x+y=w365:dbl)
        }
      }
      n105 = Bundle By Name(cluster=T6 {"dest_x"=0.0, "dest_y"=0.0, "dest_orientation"=0.0, "dest_vel"=0.0} ("element"), "dest_x"=w291, "dest_y"=w290, "dest_orientation"=w295) -> (w302:T6)
      n106 = Build Array(w302) -> (w301:T6[])
      n107 = Bundle By Name(cluster=w297, "Dest"=w301, "v_tangent"=w298, "v_normal"=w298, "v_ang"=w298, "kick_x"=0.0, "dribble"=FALSE) -> (w296:T2)
    }
  }
  "Robot out" <- w26
  n108 = feedback-in #1(w7) -> ()
  n109 = feedback-in #2(w30) -> ()
  n110 = feedback-in #3(w29) -> ()
